vi "StellarNet SpectraWiz-Chemo Globals.vi"() -> ()   [LabVIEW 2023]
panel:
  out "Detector Types":u16[](array[numeric])
  in  "Ignore error":errorcluster
  out "Y Scale.Range":T1
  in  "Chemo installed":bool
  out "Last WL":dbl
  out "1st WL":dbl
  out "WL increment":dbl
  out "Abs Data":cluster{"Wavelengths":dbl[], "Data":dbl[]}[](array[cluster])
  out "Path to model":path=path "C:/Program Files/EVRI/Solo_Predictor/application/app_bin/win32"
  out "Chemo err out":errorcluster
  in  "Chemo err in":errorcluster
  out "Chemo dll path":path=path "C:/Program Files/EVRI/Solo_Predictor/application/app_bin/win32"
  in  "Init Pending":bool
  in  "Chemo Init'd":bool
  in  "Enable Chemo":bool
  in  "Parameters file path":path
  in  "Global Stop":bool
  out "Snapshot":cluster{"Wavelengths":dbl[], sgl[]}[](array[cluster])
  out "[reference]":sgl[][](array[numeric])
  out "[dark]":sgl[][](array[numeric])
  out "Multi Channel Coeffs & WLs":T2(array[cluster])
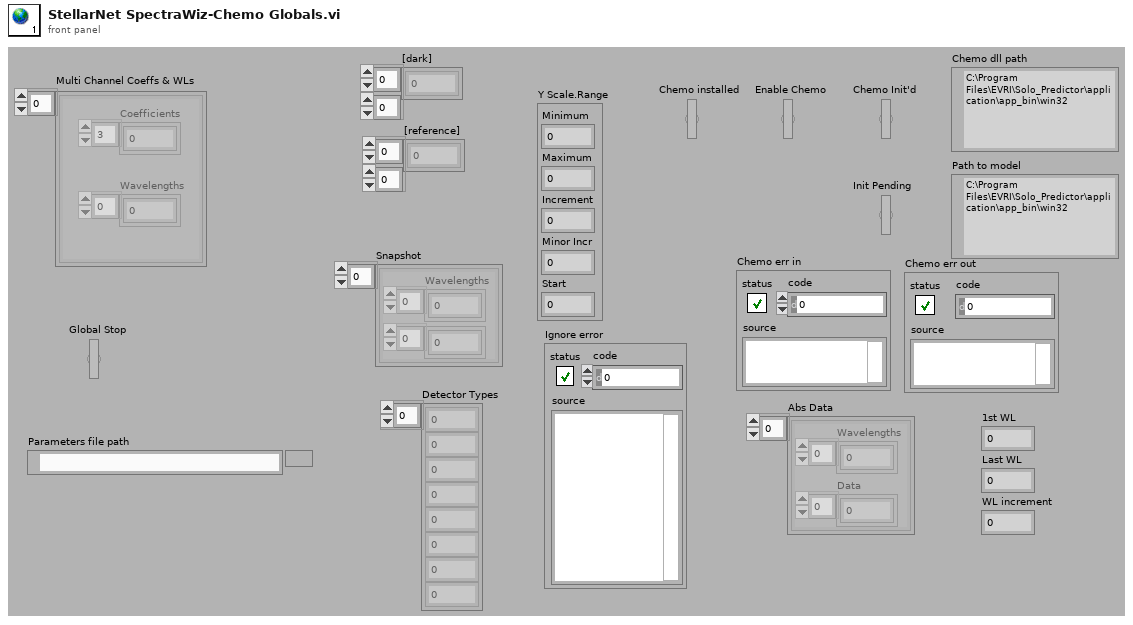
[diagram p1: front panel]
types:
  T1 = cluster{"Minimum":dbl, "Maximum":dbl, "Increment":dbl, "Minor Incr":dbl, "Start":dbl}
  T2 = cluster{"Coefficients":dbl[], "Wavelengths":dbl[]}[]
diagram:
